vi "Transpose Test Runner Error Codes.vi"(8 "error in (no error)":errorcluster, 11 "Test Runner in":refnum<class "Test Runner.lvclass">) -> (0 "error out":errorcluster, 3 "Test Runner out":refnum<class "Test Runner.lvclass">)   [LabVIEW 2013, in "Caraya.lvlib" / "Test Runner.lvclass"]
uses:
  Test Runner.lvclass
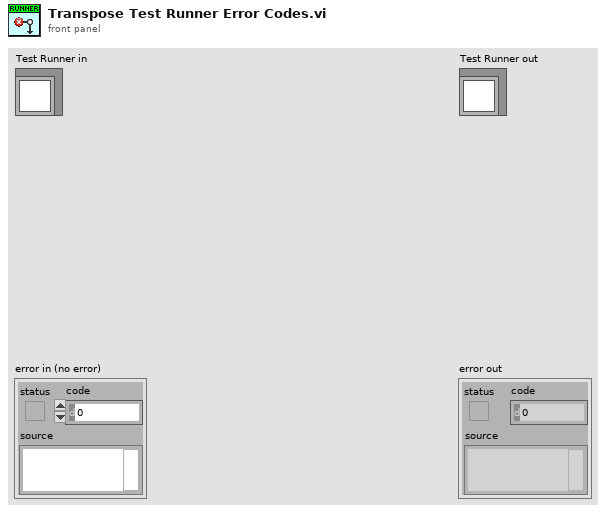
[diagram p1: front panel]
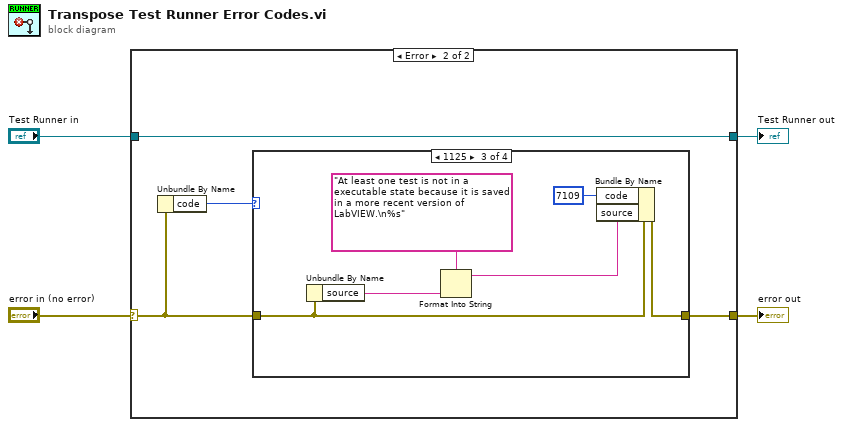
[diagram p0: block diagram]
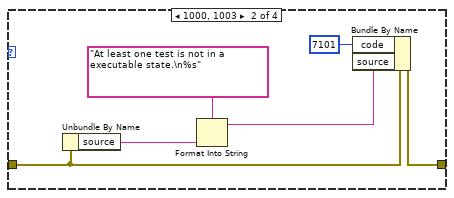
[diagram p4: hidden frame]
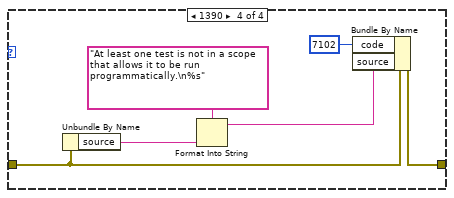
[diagram p5: hidden frame]
diagram:
  n1 = case shown="Error" "error in (no error)" {
    selector: "error in (no error)" -> [w5 w8]
    tunnel: [w5 w7] -> w3
    tunnel: [w6 w9] -> w1
    tunnel: "Test Runner in" -> [w6 w9]
    frame No Error {
    }
    frame Error {
      n2 = Unbundle By Name(w8) -> ("code"=w10:i32)
      n3 = case shown="1125" w10 {
        tunnel: w8 -> [w11 w15 w21 w27]
        tunnel: [w11 w17 w23 w29] -> w7
        frame Default {
        }
        frame 1000, 1003 {
          n4 = Unbundle By Name(w15) -> ("source"=w14:string)
          n5 = Format Into String(format string="At least one test is not in a executable state.\n%s", w14) -> (resulting string=w13:string)  [unwired: 2 in, 1 out]
          n6 = Bundle By Name(cluster=w15, "code"=7101, "source"=w13) -> (w17:errorcluster)
        }
        frame 1125 {
          n7 = Unbundle By Name(w21) -> ("source"=w20:string)
          n8 = Format Into String(format string="At least one test is not in a executable state because it is saved in a more recent version of LabVIEW.\n%s", w20) -> (resulting string=w19:string)  [unwired: 2 in, 1 out]
          n9 = Bundle By Name(cluster=w21, "code"=7109, "source"=w19) -> (w23:errorcluster)
        }
        frame 1390 {
          n10 = Unbundle By Name(w27) -> ("source"=w26:string)
          n11 = Format Into String(format string="At least one test is not in a scope that allows it to be run programmatically.\n%s", w26) -> (resulting string=w25:string)  [unwired: 2 in, 1 out]
          n12 = Bundle By Name(cluster=w27, "code"=7102, "source"=w25) -> (w29:errorcluster)
        }
      }
    }
  }
  "error out" <- w3
  "Test Runner out" <- w1
